vi "ConvertDcafUutResult.vi"(11 "UUT Result":string) -> (3 "Systemlink Status":T1=enum."None")   [LabVIEW 2018, in "TestMonitor.lvclass"]
uses:
  TestMonitor.lvclass
  <vilib>/Skyline/TestMonitor/Shared/typedefs/Status Type.ctl
  <vilib>/Skyline/TestMonitor/Shared/NI SystemLink Test Monitor.lvlib
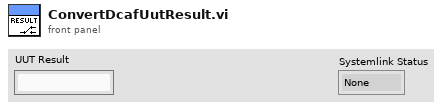
[diagram p1: front panel]
types:
  T1 = typedef "NI SystemLink Test Monitor.lvlib/Status Type.ctl" = enum16{"Failed", "Passed", "Looping", "Skipped", "Custom", "Done", "Running", "Waiting", "Terminated", "Errored", "Timed Out", "None"}
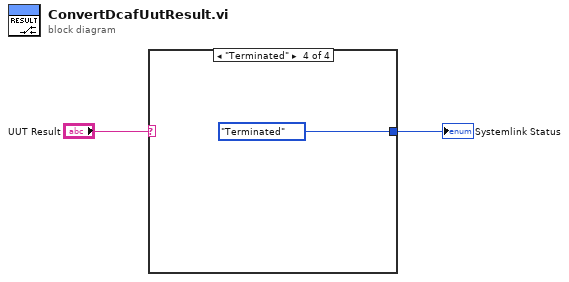
[diagram p0: block diagram]
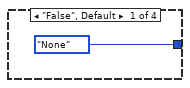
[diagram p2: hidden frame]
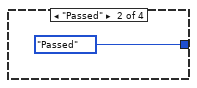
[diagram p3: hidden frame]
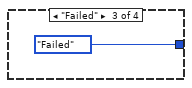
[diagram p4: hidden frame]
diagram:
  n1 = case shown="\"Terminated\"" "UUT Result" {
    tunnel: [Status_Type."None" ("Systemlink Status") Status_Type."Passed" ("Systemlink Status") Status_Type."Failed" ("Systemlink Status") Status_Type."Terminated" ("Systemlink Status")] -> w1
    frame "False", Default {
    }
    frame "Passed" {
    }
    frame "Failed" {
    }
    frame "Terminated" {
    }
  }
  "Systemlink Status" <- w1
